vi "element_editor_close.vi"(11 "Close?":bool) -> ()   [LabVIEW 2019]
panel:
  # "*******************************************************************\nBiogas Plant Control\n\nAuthor: Paul Zügel\nGCSC-Frankfurt am Main 2020\n\n*******************************************************************"
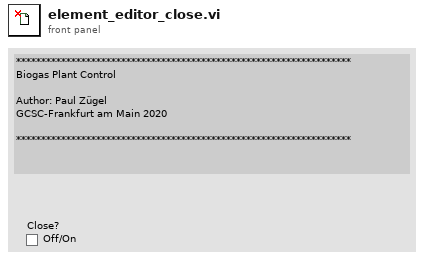
[diagram p1: front panel]
types:
  T1 = enum32{"Invalid", "Standard", "Closed", "Hidden", "Minimized", "Maximized"}
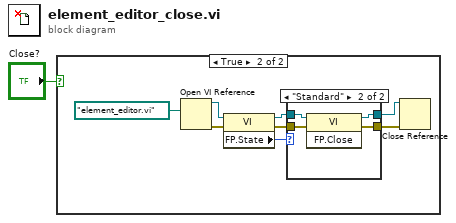
[diagram p0: block diagram]
diagram:
  n1 = case shown="True" "Close?" {
    frame False {
    }
    frame True {
      n2 = Open VI Reference(vi path=path "element_editor.vi") -> (vi reference=w5:refnum<vi>, error out=w4:errorcluster)  [unwired: 5 in]
      n3 = property class="VI"(reference=w5, error in=w4) -> (reference out=w7:refnum<vi>, error out=w6:errorcluster, "FP.State"=w8:T1)
      n4 = case shown="\"Standard\"" w8 {
        tunnel: w7 -> [w11 w15]
        tunnel: w6 -> [w10 w14]
        tunnel: [w11 w13] -> w3
        tunnel: [w10 w12] -> w2
        frame "Invalid", Default {
        }
        frame "Standard" {
          n5 = invoke class="VI" method="FP.Close"(reference=w15, error in=w14) -> (reference out=w13:refnum<vi>, error out=w12:errorcluster)  [unwired: 1 in, 1 out]
        }
      }
      n6 = Close Reference(reference=w3, error in (no error)=w2) -> ()  [unwired: 1 out]
    }
  }
